vi "GetShiftRegisters.vi"(6 "error in":errorcluster, 9 "Loop in":refnum<class "Loop.lvclass">) -> (0 "error out":errorcluster, 3 "Loop out":refnum<class "Loop.lvclass">, 4 "shift registers":i32[](array[numeric]))   [LabVIEW 2014, in "Loop.lvclass"]
uses:
  Loop.lvclass
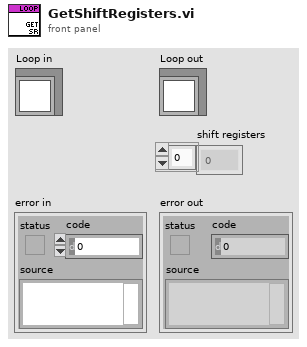
[diagram p1: front panel]
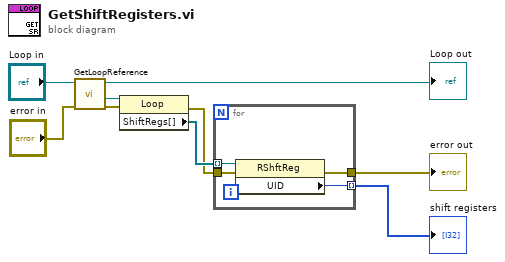
[diagram p0: block diagram]
diagram:
  n1 = call "GetLoopReference.vi"("error in"="error in", "Loop in"="Loop in") -> ("error out"=w6:errorcluster, "reference out"=w7:refnum<vi>, "Loop out"=→"Loop out":refnum<class "Loop.lvclass">)  [unwired: 7 in]
  n2 = property class="Loop"(reference=w7, error in=w6) -> (error out=w3:errorcluster, "ShiftRegs[]"=w4:refnum<vi>[])  [unwired: 1 out]
  n3 = for {
    tunnel: w4 -> [w13] mode=indexing
    tunnel: w3 -> [w12]
    tunnel: [w11] -> w1 mode=indexing
    tunnel: [w10] -> w2
    n4 = property class="RShftReg"(reference=w13, error in=w12) -> (error out=w10:errorcluster, "UID"=w11:i32)  [unwired: 1 out]
  }
  "error out" <- w2
  "shift registers" <- w1
